vi "Read Pulse Controller Configuration.vi"(8 "error in (no error)":errorcluster, 11 "Pulse Controller in":refnum<class "Pulse Controller.lvclass">) -> (0 "error out":errorcluster, 2 "Configuration":T1={"Pre-trigger duration"=-1.0, "Post-trigger duration"=-1.0, "Open plot after pulse"=FALSE, "Auto-rearm"=FALSE} {"Pre-trigger duration" format="%#_6p"; "Post-trigger duration" format="%#_6p"}, 3 "Pulse Controller out":refnum<class "Pulse Controller.lvclass">)   [LabVIEW 2018, in "Pulse Controller.lvclass"]
uses:
  Pulse Controller.lvclass
  C:/github/LabActor/Template Module/Template Module.lvclass
  Pulse Controller Configuration.ctl
  Template Module/Template Module.lvclass/Template Module.ctl
  Template Module/Read Configuration.vi
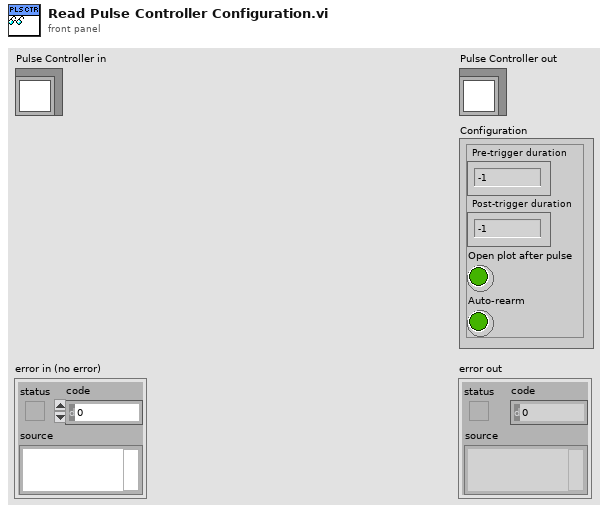
[diagram p1: front panel]
types:
  T1 = typedef "Pulse Controller Configuration.ctl" = cluster{"Pre-trigger duration":dbl, "Post-trigger duration":dbl, "Open plot after pulse":bool, "Auto-rearm":bool}
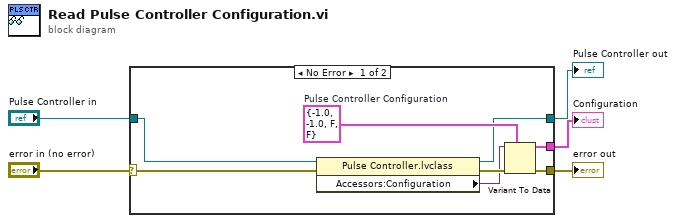
[diagram p0: block diagram]
diagram:
  n1 = case shown="No Error" "error in (no error)" {
    selector: "error in (no error)" -> [w8 w14]
    tunnel: [w9 w14] -> w4
    tunnel: [w6 w15] -> w2
    tunnel: "Pulse Controller in" -> [w7 w15]
    tunnel: [w10 _] -> w1
    frame No Error {
      w11 = T1 {"Pre-trigger duration"=-1.0, "Post-trigger duration"=-1.0, "Open plot after pulse"=FALSE, "Auto-rearm"=FALSE}  # Pulse Controller Configuration
      n2 = property class="Pulse Controller.lvclass"(reference=w7, error in=w8) -> (reference out=w6:refnum<class "Pulse Controller.lvclass">, error out=w13:errorcluster, "Accessors:Configuration"=w12:variant)
      n3 = Variant To Data(error in=w13, type=w11, Variant=w12) -> (data=w10:T1, error out=w9:errorcluster)
    }
    frame Error {
    }
  }
  "error out" <- w4
  "Pulse Controller out" <- w2
  "Configuration" <- w1
